vi "ASCII_LONG (SubVI).vi"(1 "ascii in":string) -> (0 "String out":string)   [LabVIEW 8.6]
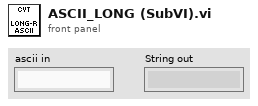
[diagram p1: front panel]
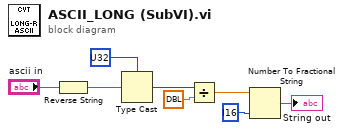
[diagram p0: block diagram]
diagram:
  n1 = Reverse String(1:"ascii in") -> (0:w7:string)
  n2 = Type Cast(type=u32 ?, x=w7) -> (*(type *) &x=w3:u32)
  n3 = Divide(x=w3, y=dbl ?) -> (x/y=w5:dbl)
  n4 = Number To Fractional String(number=w5, precision (6)=i16 ?) -> (F-format string=→"String out":string)  [unwired: 2 in]
